vi "Read Bacta [l].vi"(8 "error in (no error)":errorcluster, 11 "BactaTank in":refnum<class "BactaTank.lvclass">) -> (0 "error out":errorcluster, 2 "Bacta [l]":u8 max=100, 3 "BactaTank out":refnum<class "BactaTank.lvclass">)   [LabVIEW 2021, in "BactaTank.lvclass"]
uses:
  BactaTank.lvclass
  BactaTank.lvclass/BactaTank.ctl
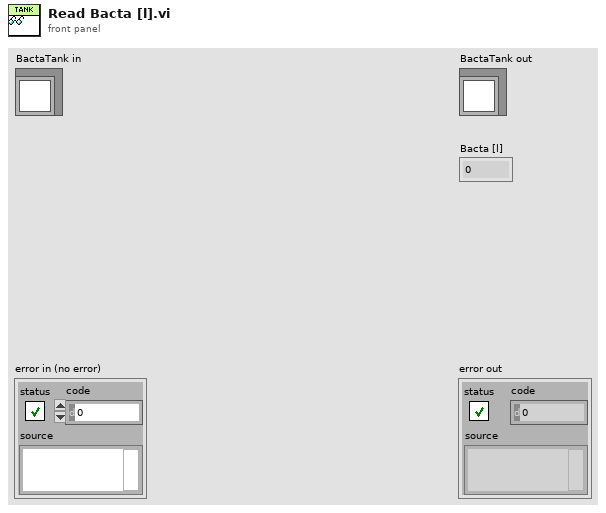
[diagram p1: front panel]
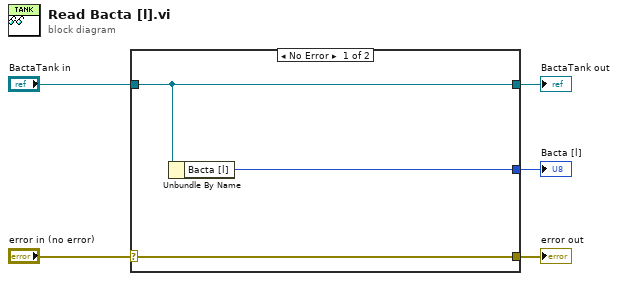
[diagram p0: block diagram]
diagram:
  n1 = case shown="No Error" "error in (no error)" {
    selector: "error in (no error)" -> [w8 w9]
    tunnel: [w8 w9] -> w4
    tunnel: [w7 w10] -> w2
    tunnel: "BactaTank in" -> [w7 w10]
    tunnel: [w6 _] -> w1
    frame No Error {
      n2 = Unbundle By Name(w7) -> ("Bacta [l]"=w6:u8)
    }
    frame Error {
    }
  }
  "error out" <- w4
  "BactaTank out" <- w2
  "Bacta [l]" <- w1
